vi "Insert TSC tEXt Chunk.vi"(1 "png binary string":string) -> (0 "New PNG Binary":u8[](array[numeric]) format="%.0x")   [LabVIEW 2021, in "TSC Material Theme.lvlib" / "Material-Scheme.lvclass"]
doc: "embed the png author text chunk into the image\n\n<b>Code Developed By:</b>\nTechnology Service Corporation\nwww.tsc.com/atcs\n\nDeveloper:\nDaniel Coons"
uses:
  Material-Scheme.lvclass
  Material-Scheme.lvclass/Material-Scheme.ctl
panel:
  out "output binary string":string
  out "appended array":u8[](array[numeric])
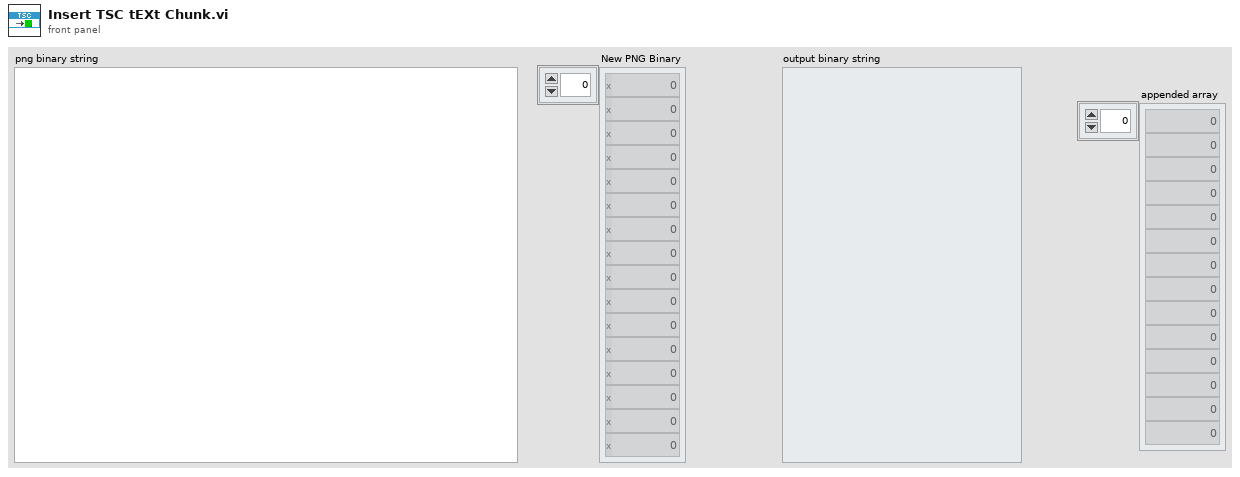
[diagram p1: front panel]
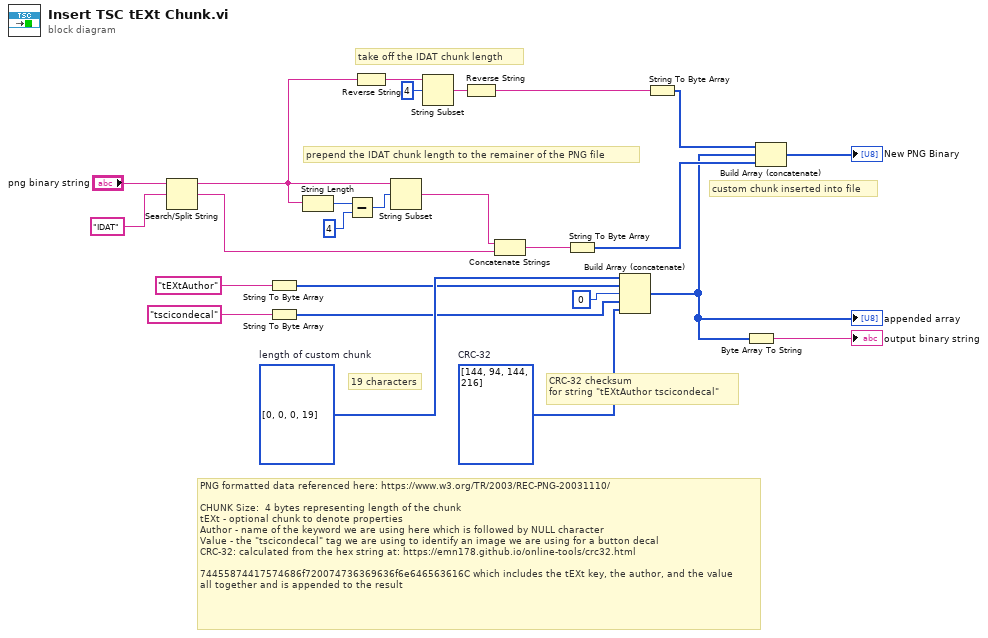
[diagram p0: block diagram]
diagram:
  w23 = u8[] [0, 0, 0, 19]  # length of custom chunk
  w24 = u8[] [144, 94, 144, 216]  # CRC-32
  # "custom chunk inserted into file"
  # "CRC-32 checksum\nfor string \"tEXtAuthor tscicondecal\""
  # "19 characters"
  # "prepend the IDAT chunk length to the remainer of the PNG file"
  # "take off the IDAT chunk length"
  # "PNG formatted data referenced here: https://www.w3.org/TR/2003/REC-PNG-20031110/\n\nCHUNK Size:  4 bytes representing length of the chunk\ntEXt - optional chunk to denote properties\nAuthor - name of the keyword we are using here which is followed by NULL character\nValue - the \"tscicondecal\" tag we are using to identify an image we are using for a button decal\nCRC-32: calculated from the hex string at: https://emn178.github.io/online-tools/crc32.html\n\n74455874417574686f720074736369636f6e646563616C which includes the tEXt key, the author, and the value\nall together and is appended to the result"
  n1 = Search/Split String(string="png binary string", search string/char (-)="IDAT") -> (substring before match=w18:string, match + rest of string=w20:string)  [unwired: 1 in, 1 out]
  n2 = String To Byte Array(string="tEXtAuthor") -> (unsigned byte array=w8:u8[])
  n3 = String To Byte Array(string="tscicondecal") -> (unsigned byte array=w9:u8[])
  n4 = String Length(string=w18) -> (length=w12:i32)
  n5 = Subtract(x=w12, y=4) -> (x-y=w15:i32)
  n6 = Reverse String(1:w18) -> (0:w14:string)
  n7 = String Subset(string=w18, offset (0)=w15) -> (substring=w19:string)  [unwired: 1 in]
  n8 = String Subset(string=w14, offset (0)=4) -> (substring=w16:string)  [unwired: 1 in]
  n9 = Reverse String(1:w16) -> (0:w22:string)
  n10 = Concatenate Strings(w19, w20) -> (w21:string)
  n11 = String To Byte Array(string=w21) -> (unsigned byte array=w6:u8[])
  n12 = Build Array (concatenate)(w23, w8, u8 0, w9, w24) -> (w2:u8[])
  "appended array" <- w2
  n13 = String To Byte Array(string=w22) -> (unsigned byte array=w4:u8[])
  n14 = Byte Array To String(unsigned byte array=w2) -> (string=→"output binary string":string)
  n15 = Build Array (concatenate)(w4, w2, w6) -> (→"New PNG Binary":u8[])
